vi "Bundle_N_Data.vi"(0 "Data_Type":T1, 5 "Parent":string, 9 "Children_Names":string[](array[string])) -> (4 "Data_Out":T1[](array[typedef]))   [LabVIEW 2021]
uses:
  Controls/State_and_Data.ctl
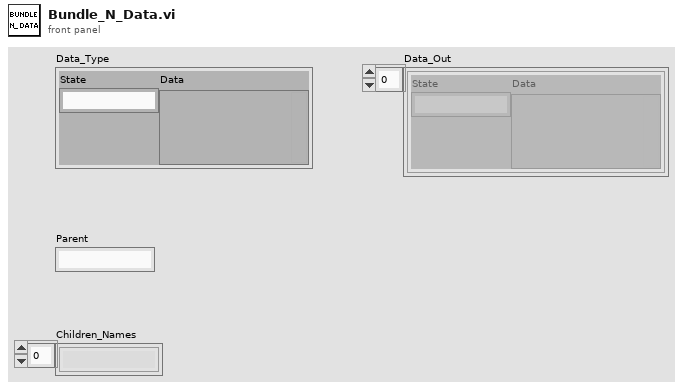
[diagram p1: front panel]
types:
  T1 = typedef "State_and_Data.ctl" = cluster{"State":string, "Data":variant}
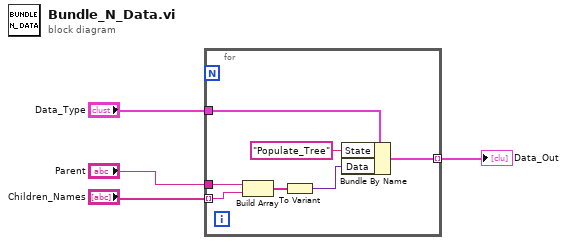
[diagram p0: block diagram]
diagram:
  n1 = for {
    tunnel: "Children_Names" -> [w9] mode=indexing
    tunnel: "Parent" -> [w10]
    tunnel: [w6] -> w3 mode=indexing
    tunnel: "Data_Type" -> [w5]
    n2 = Build Array(w10, w9) -> (w8:string[])
    n3 = To Variant(anything=w8) -> (Variant=w7:variant)
    n4 = Bundle By Name(cluster=w5, "State"="Populate_Tree", "Data"=w7) -> (w6:T1)
  }
  "Data_Out" <- w3
